vi "CallByRefParallel Set control values.vi"(8 "error in (no error)":errorcluster, 9 "Control values":variant[](array[variant]), 10 "Control names":string[](array[string]), 11 "VI Refnum":refnum<vi>) -> (0 "error out":errorcluster, 3 "VI Refnum dup":refnum<vi>)   [LabVIEW 2014, in "COSYLib.lvlib"]
doc: "Simple wrapper around a series of \"Set Control Value\" (Ctrl Val.Set) calls for a target VI."
uses:
  COSYLib.lvlib
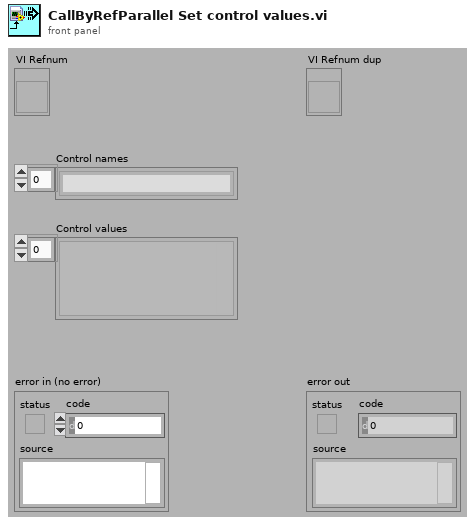
[diagram p1: front panel]
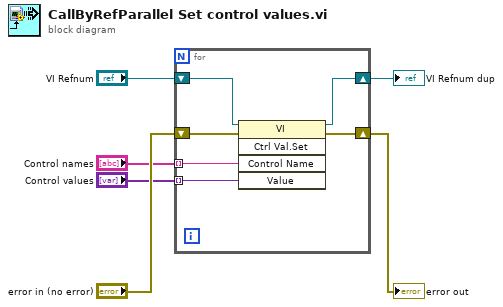
[diagram p0: block diagram]
diagram:
  n1 = for {
    shift-right: [w11] -> w5
    shift-left: "VI Refnum" -> [w12]
    tunnel: "Control names" -> [w10] mode=indexing
    tunnel: "Control values" -> [w9] mode=indexing
    shift-right: [w7] -> w1
    shift-left: "error in (no error)" -> [w8]
    n2 = invoke class="VI" method="Ctrl Val.Set"(reference=w12, error in=w8, "Control Name"=w10, "Value"=w9) -> (reference out=w11:refnum<vi>, error out=w7:errorcluster)  [unwired: 1 in, 3 out]
  }
  "VI Refnum dup" <- w5
  "error out" <- w1
